vi "Start Widget Engine.vi"(8 "Error In":errorcluster) -> (0 "Error Out":errorcluster)   [LabVIEW 2013, in "Template.lvlib" / "LQWidgetEngine.lvclass"]
uses:
  LQWidgetEngine.lvclass
  Private/Global Quit Event Holder.vi
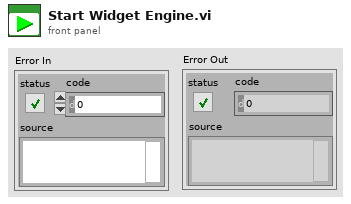
[diagram p1: front panel]
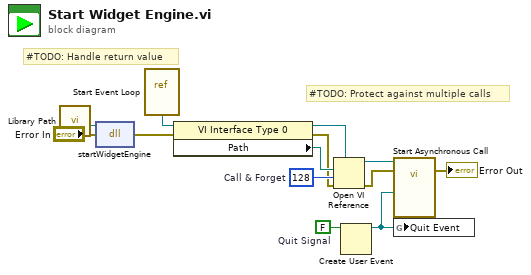
[diagram p0: block diagram]
diagram:
  w10 = 128  # Call & Forget
  w12 = FALSE  # Quit Signal
  # "#TODO: Protect against multiple calls"
  # "#TODO: Handle return value"
  n1 = call "Library Path.vi"() -> ("Library Path"=w1:path)
  n2 = dll-call lib="?" fn="startWidgetEngine"(path in=w1, error in="Error In") -> (error out=w5:errorcluster)  [unwired: 2 in, 1 out]
  n3 = vi-ref "Start Event Loop.vi"() -> (w7:refnum<vi>)
  n4 = property class="VI Interface Type 0"(reference=w7, error in=w5) -> (reference out=w8:refnum<vi>, error out=w4:errorcluster, "Path"=w9:path)
  n5 = Open VI Reference(type specifier VI Refnum (for type only)=w8, vi path=w9, options=w10, error in (no error)=w4) -> (vi reference=w6:refnum<vi>, error out=w3:errorcluster)  [unwired: 2 in]
  n6 = Create User Event(user event datatype=w12) -> (user event=w11:refnum<user-event>)  [unwired: 1 in, 1 out]
  n7 = call-by-ref "Start Asynchronous Call"(reference=w6, error in=w3, "Quit Event"=w11) -> (error out=→"Error Out":errorcluster)  [unwired: 11 in, 1 out]
  n8 = global write "Global Quit Event Holder.vi" "Quit Event"(w11) -> ()
